vi "Stop Fire.vi"(9 "Height":i32, 10 "Width":i32, 11 "Pixel Array In":i32[](array[numeric])) -> (3 "Pixel Array Out":i32[](array[numeric]))   [LabVIEW 2018]
doc: "Removes the fire source by randomly decreasing its intensity until it is removed completely. Repeated calls to Do Fire.vi will then burn up the remainder of the fire."
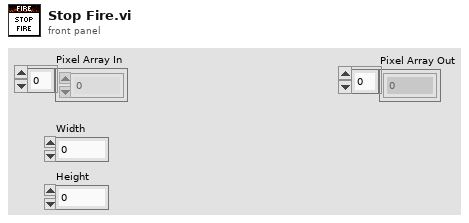
[diagram p1: front panel]
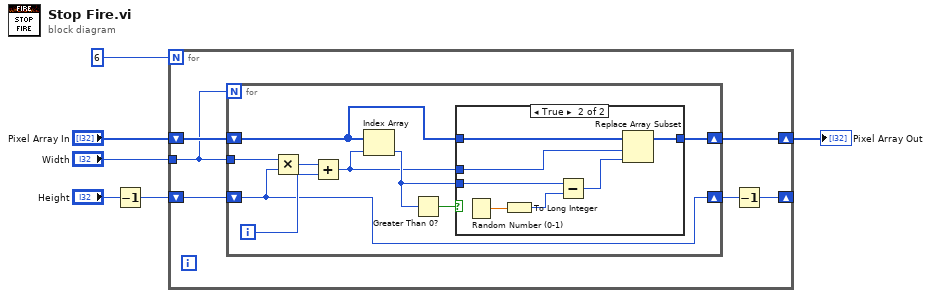
[diagram p0: block diagram]
diagram:
  n1 = Decrement(x="Height") -> (x-1=w1:i32)
  n2 = for {
    N: 6 -> [_]
    shift-right: [w11] -> w5
    shift-left: "Pixel Array In" -> [w12]
    tunnel: "Width" -> [w10]
    shift-right: [w9] -> _
    shift-left: w1 -> [w8]
    n3 = for {
      N: w10 -> [_]
      shift-right: [w17] -> w11
      shift-left: w12 -> [w16]
      tunnel: w10 -> [w21]
      shift-right: [w13] -> w7
      shift-left: w8 -> [w13]
      i -> [w19]
      n4 = Multiply(x=w21, y=w13) -> (x*y=w20:i32)
      n5 = Add(x=w20, y=w19) -> (x+y=w14:i32)
      n6 = Index Array(array=w16, index=w14) -> (element=w15:i32)
      n7 = Greater Than 0?(x=w15) -> (x > 0?=w18:bool)
      n8 = case shown="True" w18 {
        tunnel: [w22 w28] -> w17
        tunnel: w16 -> [w22 w29]
        tunnel: w15 -> [_ w26]
        tunnel: w14 -> [_ w25]
        frame False {
        }
        frame True {
          n9 = Random Number (0-1)() -> (number: 0 to 1=w27:dbl)
          n10 = To Long Integer(number=w27) -> (32bit integer=w24:i32)
          n11 = Subtract(x=w26, y=w24) -> (x-y=w23:i32)
          n12 = Replace Array Subset(array=w29, new element=w23, index=w25) -> (w28:i32[])
        }
      }
    }
    n13 = Decrement(x=w7) -> (x-1=w9:i32)
  }
  "Pixel Array Out" <- w5
